vi "ex3-1.vi"() -> ()   [LabVIEW 2009]
panel:
  out "X+Y":dbl
  in  "Y":dbl
  in  "X":dbl
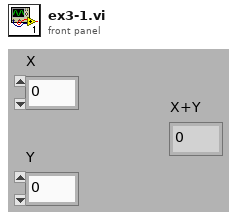
[diagram p1: front panel]
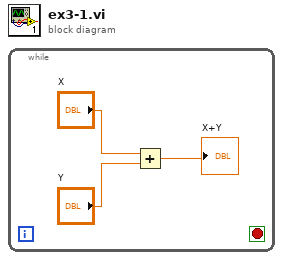
[diagram p0: block diagram]
diagram:
  n1 = while {
    stop <- _ stop-if-true
    n2 = Add(x="X", y="Y") -> (x+y=→"X+Y":dbl)
  }
